vi "Insert Step at Index.vi"(8 "error in (no error)":errorcluster, 9 "Element":i32, 10 "Step":refnum<class "Base Step.lvclass">, 11 "Loop in":refnum<class "Loop.lvclass">) -> (0 "error out":errorcluster, 3 "Loop out":refnum<class "Loop.lvclass">)   [LabVIEW 2024, in "Ramses Sequencer.lvlib" / "Loop.lvclass"]
uses:
  Loop.lvclass
  Base Step/Base Step.lvclass
  Loop.lvclass/Loop.ctl
  Sequence/Sequence.lvclass
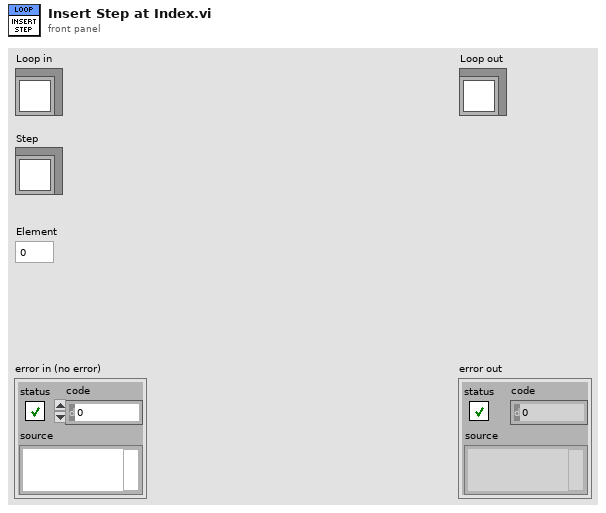
[diagram p1: front panel]
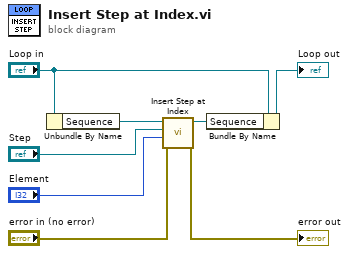
[diagram p0: block diagram]
diagram:
  n1 = Unbundle By Name("Loop in") -> ("Sequence"=w6:refnum<class "Sequence.lvclass">)
  n2 = call "Insert Step at Index.vi"("error in (no error)"="error in (no error)", "Index"="Element", "Step"="Step", "Sequence in"=w6) -> ("error out"=→"error out":errorcluster, "Sequence out"=w5:refnum<class "Sequence.lvclass">)  [unwired: 6 in]
  n3 = Bundle By Name(cluster="Loop in", "Sequence"=w5) -> (→"Loop out":refnum<class "Loop.lvclass">)
